vi "ReadPAQdata.vi"(4 "Tags":string[](array[string]), 6 "TableName":string, 8 "error in (no error)":errorcluster, 9 "Time-End":timestamp, 10 "Time-Start":timestamp, 11 "DBAL-BIN in":refnum<class "DBAL-BIN.lvclass">) -> (0 "error out":errorcluster, 2 "PAQ_section":T1, 3 "DBAL-BIN out":refnum<class "DBAL-BIN.lvclass">)   [LabVIEW 2020, in "Sgraph_lib_V1.lvlib" / "DBAL-BIN.lvclass"]
doc: "Andre Koelewijn, 8 May 2021,\n\nRead a PAQ TAGs from the BIN database for a defined time span.\nThe Layer input defines from which layer the data should be read.\nRev 1, 16 nov 2021, fixed gap when passing a day (midnight)"
uses:
  DBAL-BIN.lvclass
  controls/BIN/BINdata.ctl
  DBAL-BIN.lvclass/DBAL-BIN.ctl
  Gview/Gviewer.lvclass
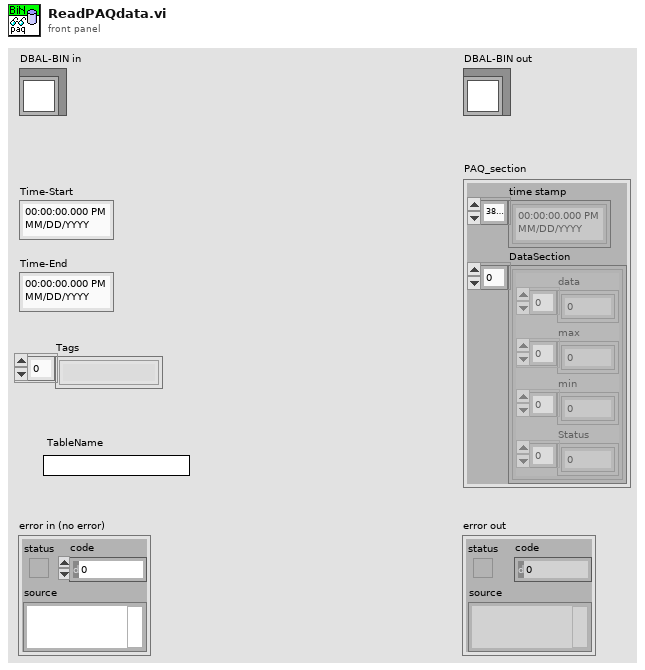
[diagram p1: front panel]
types:
  T1 = cluster{"time stamp":timestamp[], "DataSection":cluster{"data":dbl[], "max":dbl[], "min":dbl[], "Status":u32[]}[]}
  T2 = typedef "Sgraph_lib_V1.lvlib/DBAL-BIN.lvclass/BINdata.ctl" = cluster{"time":dbl[], "TagsData":cluster{"data":dbl[], "max":dbl[], "min":dbl[], "status":u32[]}[]}
  T3 = typedef "Sgraph_lib_V1.lvlib/DBAL-BIN.lvclass/BinFolderPace.ctl" = enum16{"PerDay", "PerWeek", "PerYear"}
  T4 = cluster{"Seq":i32, "Start":timestamp, "Stop":timestamp, "table":string}[]
  T5 = cluster{"data":dbl[], "max":dbl[], "min":dbl[], "status":u32[]}[]
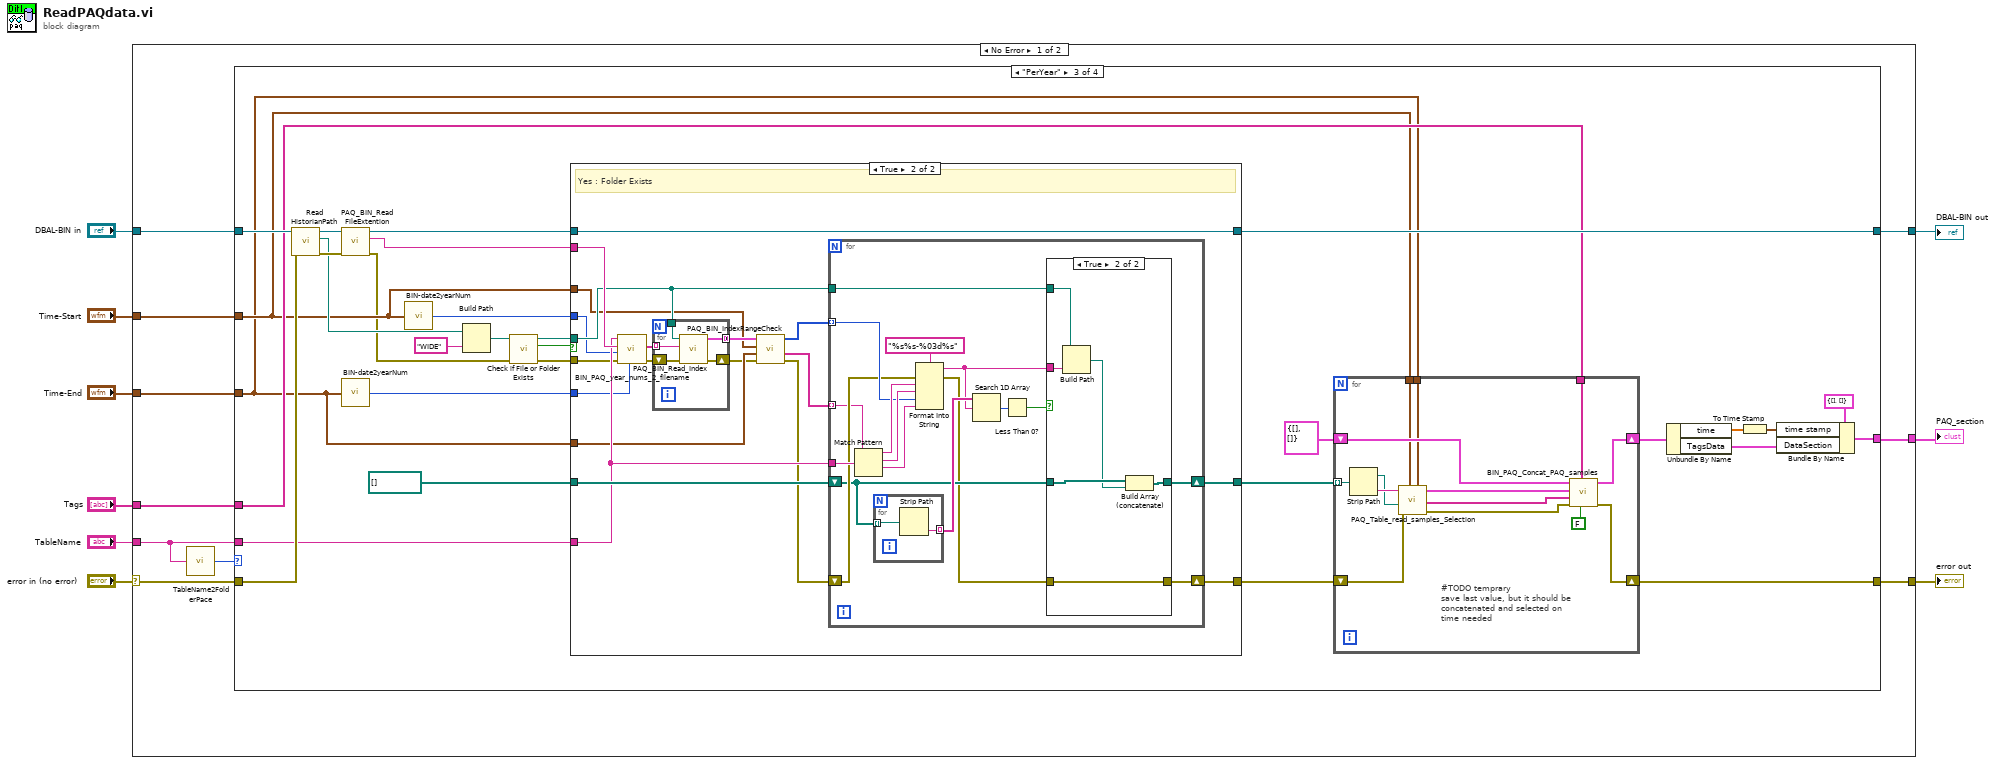
[diagram p0: block diagram]
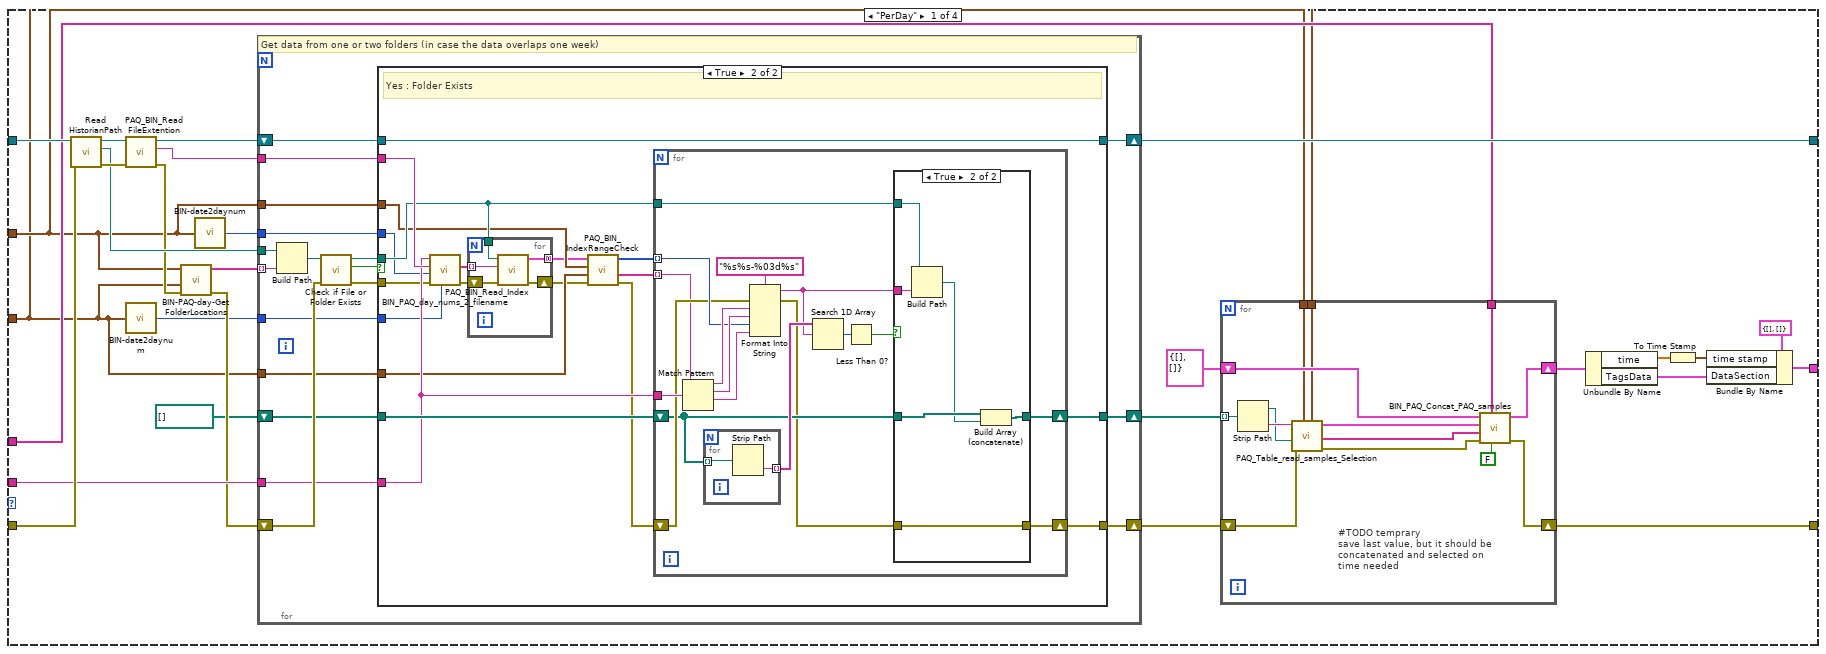
[diagram p2: hidden frame]
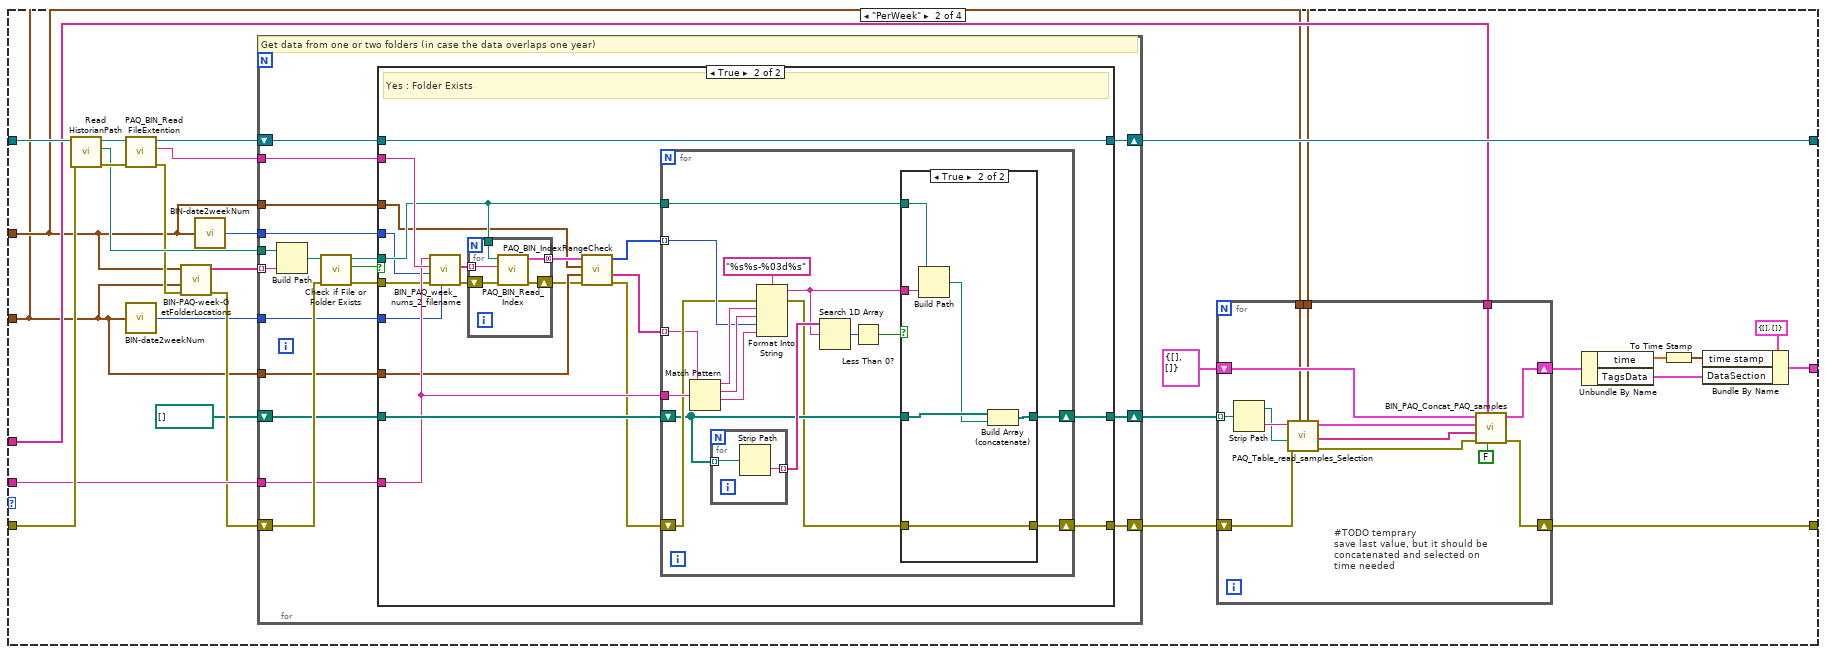
[diagram p5: hidden frame]
diagram:
  n1 = case shown="No Error" "error in (no error)" {
    selector: "error in (no error)" -> [w16 w350]
    tunnel: [w15 w350] -> w8
    tunnel: [w17 w349] -> w6
    tunnel: "DBAL-BIN in" -> [w18 w349]
    tunnel: "Time-Start" -> [w13 _]
    tunnel: "Time-End" -> [w12 _]
    tunnel: "Tags" -> [w11 _]
    tunnel: "TableName" -> [w14 _]
    tunnel: [w10 _] -> w1
    frame No Error {
      n2 = call "TableName2FolderPace.vi"("TableName"=w14) -> ("FolderPace"=w19:T3)  [unwired: 6 in]
      n3 = case shown="\"PerYear\"" w19 {
        tunnel: w18 -> [w47 w161 w278 w348]
        tunnel: [w42 w156 w273 w348] -> w17
        tunnel: w16 -> [w44 w158 w275 w347]
        tunnel: [w30 w144 w264 w347] -> w15
        tunnel: w14 -> [w41 w155 w272 _]
        tunnel: w13 -> [w21 w135 w255 _]
        tunnel: w12 -> [w20 w134 w254 _]
        tunnel: w11 -> [w22 w136 w256 _]
        tunnel: [w23 w137 w257 _] -> w10
        frame "PerDay" {
          n4 = call "Read HistorianPath.vi"("error in (no error)"=w44, "DBAL-BIN in"=w47) -> ("error out"=w45:errorcluster, "HistorianPath"=w39:path, "DBAL-BIN out"=w46:refnum<class "DBAL-BIN.lvclass">)  [unwired: 7 in]
          n5 = call "PAQ_BIN_Read FileExtention.vi"("error in (no error)"=w45, "DBAL-BIN in"=w46) -> ("error out"=w38:errorcluster, "FileExtention"=w40:string, "DBAL-BIN out"=w43:refnum<class "DBAL-BIN.lvclass">)  [unwired: 7 in]
          n6 = call "BIN-date2daynum.vi"("Time"=w20) -> ("DayNum"=w33:u64)  [unwired: 8 in]
          n7 = call "BIN-PAQ-day-GetFolderLocations.vi"("error in (no error)"=w38, "Time-End"=w20, "Time-Start"=w21) -> ("error out"=w36:errorcluster, "Folders"=w37:string[])  [unwired: 6 in, 1 out]
          n8 = call "BIN-date2daynum.vi"("Time"=w21) -> ("DayNum"=w32:u64)  [unwired: 8 in]
          n9 = for {
            shift-right: [w72] -> w31
            shift-left: w36 -> [w76]
            shift-right: [w73] -> w42
            shift-left: w43 -> [w74]
            tunnel: w37 -> [w78] mode=indexing
            tunnel: w41 -> [w66]
            tunnel: w39 -> [w79]
            tunnel: w40 -> [w71]
            shift-right: [w68] -> w34
            shift-left: path[] [] -> [w67]
            tunnel: w33 -> [w64]
            tunnel: w32 -> [w65]
            tunnel: w21 -> [w63]
            tunnel: w20 -> [w62]
            # "Get data from one or two folders (in case the data overlaps one week)"
            n10 = Build Path(base path=w79, name or relative path=w78) -> (appended path=w77:path)
            n11 = call <vilib>:"Check if File or Folder Exists.vi"("error in (no error)"=w76, "path"=w77) -> ("error out"=w69:errorcluster, "file or folder exists?"=w75:bool, "dup path"=w70:path)  [unwired: 7 in]
            n12 = case shown="True" w75 {
              tunnel: w74 -> [w82 w100]
              tunnel: [w82 w100] -> w73
              tunnel: [w81 w99] -> w72
              tunnel: w71 -> [_ w101]
              tunnel: w70 -> [_ w95]
              tunnel: w69 -> [w81 w93]
              tunnel: [w80 w97] -> w68
              tunnel: w67 -> [w80 w98]
              tunnel: w66 -> [_ w96]
              tunnel: w65 -> [_ w92]
              tunnel: w64 -> [_ w91]
              tunnel: w63 -> [_ w89]
              tunnel: w62 -> [_ w88]
              frame False {
                # "No: Folder not found"
              }
              frame True {
                # "Yes : Folder Exists"
                n13 = call "BIN_PAQ_day_nums_2_filename.vi"("num Stop"=w91, "error in"=w93, "num Start"=w92, "ext"=w101, "TableName"=w96) -> ("error out"=w94:errorcluster, "FileNames"=w90:string[])  [unwired: 5 in]
                n14 = for {
                  tunnel: [w106] -> w87 mode=concatenating
                  tunnel: w95 -> [w104]
                  shift-right: [w105] -> w84
                  shift-left: w94 -> [w103]
                  tunnel: w90 -> [w102] mode=indexing
                  n15 = call "PAQ_BIN_Read_Index.vi"("error in (no error)"=w103, "TableName"=w102, "Path"=w104) -> ("error out"=w105:errorcluster, "TimeStamps"=w106:T4)  [unwired: 7 in]
                }
                n16 = call "PAQ_BIN_IndexRangeCheck.vi"("error in (no error)"=w84, "Stop"=w88, "Start"=w89, "TimeStamps"=w87) -> ("error out"=w83:errorcluster, "Tables"=w85:string[], "Sequences"=w86:i32[])  [unwired: 5 in]
                n17 = for {
                  shift-right: [w108] -> w99
                  shift-left: w83 -> [w116]
                  tunnel: w86 -> [w119] mode=indexing
                  shift-right: [w110] -> w97
                  shift-left: w98 -> [w111]
                  tunnel: w96 -> [w123]
                  tunnel: w95 -> [w112]
                  tunnel: w85 -> [w107] mode=indexing
                  n18 = Match Pattern(string=w107, regular expression=w123) -> (before substring=w121:string, match substring=w120:string, after substring=w118:string)  [unwired: 1 in, 1 out]
                  n19 = for {
                    tunnel: w111 -> [w133] mode=indexing
                    tunnel: [w132] -> w117 mode=indexing
                    n20 = Strip Path(path=w133) -> (name=w132:string)  [unwired: 1 out]
                  }
                  n21 = Format Into String(format string="%s%s-%03d%s", error in=w116, w121, w120, w119, w118) -> (resulting string=w113:string, error out=w109:errorcluster)  [unwired: 1 in]
                  n22 = Search 1D Array(1D array=w117, element=w113) -> (index of element=w115:i32)  [unwired: 1 in]
                  n23 = Less Than 0?(x=w115) -> (x < 0?=w114:bool)
                  n24 = case shown="True" w114 {
                    tunnel: w113 -> [_ w130]
                    tunnel: w112 -> [_ w131]
                    tunnel: w111 -> [w125 w127]
                    tunnel: [w125 w128] -> w110
                    tunnel: w109 -> [w124 w129]
                    tunnel: [w124 w129] -> w108
                    frame False {
                    }
                    frame True {
                      n25 = Build Path(base path=w131, name or relative path=w130) -> (appended path=w126:path)
                      n26 = Build Array (concatenate)(w127, w126) -> (w128:path[])
                    }
                  }
                }
              }
            }
          }
          n27 = for {
            tunnel: w34 -> [w60] mode=indexing
            shift-right: [w51] -> w30
            shift-left: w31 -> [w61]
            shift-right: [w56] -> w24
            shift-left: T2 {"time"=[], "TagsData"=[]} ("BinHistData") -> [w57]
            tunnel: w22 -> [w54]
            tunnel: w21 -> [w50]
            tunnel: w20 -> [w49]
            # "#TODO temprary\nsave last value, but it should be\nconcatenated and selected on \ntime needed"
            n28 = Strip Path(path=w60) -> (stripped path=w58:path, name=w59:string)
            n29 = call "PAQ_Table_read_samples_Selection.vi"("Time-End"=w49, "Time-Start"=w50, "error in (no error)"=w61, "Sub Path"=w58, "Table Filename"=w59) -> ("error out"=w52:errorcluster, "TAGs"=w53:string[], "Fetched PAQ-samples"=w55:T2)  [unwired: 3 in, 1 out]
            n30 = call "BIN_PAQ_Concat_PAQ_samples.vi"("Reversed"=FALSE, "Memory TAGs"=w54, "error in (no error)"=w52, "Added samples TAGs"=w53, "PAQ Samples to ADD"=w55, "PAQ Samples IN"=w57) -> ("error out"=w51:errorcluster, "PAQ Samples OUT"=w56:T2)  [unwired: 4 in]
          }
          n31 = Unbundle By Name(w24) -> ("time"=w27:dbl[], "TagsData"=w28:T5)
          n32 = To Time Stamp(1:w27) -> (0:w26:timestamp[])
          n33 = Bundle By Name(cluster=T1 {"time stamp"=[], "DataSection"=[]} ("PAQ_section"), "time stamp"=w26, "DataSection"=w28) -> (w23:T1)
        }
        frame "PerWeek" {
          n34 = call "Read HistorianPath.vi"("error in (no error)"=w158, "DBAL-BIN in"=w161) -> ("error out"=w159:errorcluster, "HistorianPath"=w153:path, "DBAL-BIN out"=w160:refnum<class "DBAL-BIN.lvclass">)  [unwired: 7 in]
          n35 = call "PAQ_BIN_Read FileExtention.vi"("error in (no error)"=w159, "DBAL-BIN in"=w160) -> ("error out"=w152:errorcluster, "FileExtention"=w154:string, "DBAL-BIN out"=w157:refnum<class "DBAL-BIN.lvclass">)  [unwired: 7 in]
          n36 = call "BIN-date2weekNum.vi"("Time"=w134) -> ("WeekNum"=w147:u64)  [unwired: 8 in]
          n37 = call "BIN-PAQ-week-GetFolderLocations.vi"("error in (no error)"=w152, "Time-End"=w134, "Time-Start"=w135) -> ("error out"=w150:errorcluster, "Folders"=w151:string[])  [unwired: 6 in, 1 out]
          n38 = call "BIN-date2weekNum.vi"("Time"=w135) -> ("WeekNum"=w146:u64)  [unwired: 8 in]
          n39 = for {
            shift-right: [w186] -> w145
            shift-left: w150 -> [w190]
            shift-right: [w187] -> w156
            shift-left: w157 -> [w188]
            tunnel: w151 -> [w192] mode=indexing
            tunnel: w155 -> [w180]
            tunnel: w153 -> [w193]
            tunnel: w154 -> [w185]
            shift-right: [w182] -> w148
            shift-left: path[] [] -> [w181]
            tunnel: w147 -> [w178]
            tunnel: w146 -> [w179]
            tunnel: w135 -> [w177]
            tunnel: w134 -> [w176]
            # "Get data from one or two folders (in case the data overlaps one year)"
            n40 = Build Path(base path=w193, name or relative path=w192) -> (appended path=w191:path)
            n41 = call <vilib>:"Check if File or Folder Exists.vi"("error in (no error)"=w190, "path"=w191) -> ("error out"=w183:errorcluster, "file or folder exists?"=w189:bool, "dup path"=w184:path)  [unwired: 7 in]
            n42 = case shown="True" w189 {
              tunnel: w188 -> [w196 w214]
              tunnel: [w196 w214] -> w187
              tunnel: [w195 w213] -> w186
              tunnel: w185 -> [_ w215]
              tunnel: w184 -> [_ w209]
              tunnel: w183 -> [w195 w207]
              tunnel: [w194 w211] -> w182
              tunnel: w181 -> [w194 w212]
              tunnel: w180 -> [_ w210]
              tunnel: w179 -> [_ w206]
              tunnel: w178 -> [_ w205]
              tunnel: w177 -> [_ w202]
              tunnel: w176 -> [_ w201]
              frame False {
                # "No: Folder not found"
              }
              frame True {
                # "Yes : Folder Exists"
                n43 = call "BIN_PAQ_week_nums_2_filename.vi"("num Stop"=w205, "error in"=w207, "num Start"=w206, "ext"=w215, "TableName"=w210) -> ("error out"=w208:errorcluster, "FileNames"=w204:string[])  [unwired: 5 in]
                n44 = for {
                  tunnel: [w220] -> w203 mode=concatenating
                  tunnel: w209 -> [w218]
                  shift-right: [w219] -> w200
                  shift-left: w208 -> [w217]
                  tunnel: w204 -> [w216] mode=indexing
                  n45 = call "PAQ_BIN_Read_Index.vi"("error in (no error)"=w217, "TableName"=w216, "Path"=w218) -> ("error out"=w219:errorcluster, "TimeStamps"=w220:T4)  [unwired: 7 in]
                }
                n46 = call "PAQ_BIN_IndexRangeCheck.vi"("error in (no error)"=w200, "Stop"=w201, "Start"=w202, "TimeStamps"=w203) -> ("error out"=w199:errorcluster, "Tables"=w197:string[], "Sequences"=w198:i32[])  [unwired: 5 in]
                n47 = for {
                  shift-right: [w222] -> w213
                  shift-left: w199 -> [w230]
                  tunnel: w198 -> [w233] mode=indexing
                  shift-right: [w224] -> w211
                  shift-left: w212 -> [w225]
                  tunnel: w210 -> [w237]
                  tunnel: w209 -> [w226]
                  tunnel: w197 -> [w221] mode=indexing
                  n48 = Match Pattern(string=w221, regular expression=w237) -> (before substring=w235:string, match substring=w234:string, after substring=w232:string)  [unwired: 1 in, 1 out]
                  n49 = for {
                    tunnel: w225 -> [w247] mode=indexing
                    tunnel: [w246] -> w231 mode=indexing
                    n50 = Strip Path(path=w247) -> (name=w246:string)  [unwired: 1 out]
                  }
                  n51 = Format Into String(format string="%s%s-%03d%s", error in=w230, w235, w234, w233, w232) -> (resulting string=w227:string, error out=w223:errorcluster)  [unwired: 1 in]
                  n52 = Search 1D Array(1D array=w231, element=w227) -> (index of element=w229:i32)  [unwired: 1 in]
                  n53 = Less Than 0?(x=w229) -> (x < 0?=w228:bool)
                  n54 = case shown="True" w228 {
                    tunnel: w227 -> [_ w244]
                    tunnel: w226 -> [_ w245]
                    tunnel: w225 -> [w239 w242]
                    tunnel: [w239 w240] -> w224
                    tunnel: w223 -> [w238 w243]
                    tunnel: [w238 w243] -> w222
                    frame False {
                    }
                    frame True {
                      n55 = Build Path(base path=w245, name or relative path=w244) -> (appended path=w241:path)
                      n56 = Build Array (concatenate)(w242, w241) -> (w240:path[])
                    }
                  }
                }
              }
            }
          }
          n57 = for {
            tunnel: w148 -> [w174] mode=indexing
            shift-right: [w165] -> w144
            shift-left: w145 -> [w175]
            shift-right: [w170] -> w138
            shift-left: T2 {"time"=[], "TagsData"=[]} ("BinHistData") -> [w171]
            tunnel: w136 -> [w168]
            tunnel: w135 -> [w164]
            tunnel: w134 -> [w163]
            # "#TODO temprary\nsave last value, but it should be\nconcatenated and selected on \ntime needed"
            n58 = Strip Path(path=w174) -> (stripped path=w172:path, name=w173:string)
            n59 = call "PAQ_Table_read_samples_Selection.vi"("Time-End"=w163, "Time-Start"=w164, "error in (no error)"=w175, "Sub Path"=w172, "Table Filename"=w173) -> ("error out"=w166:errorcluster, "TAGs"=w167:string[], "Fetched PAQ-samples"=w169:T2)  [unwired: 3 in, 1 out]
            n60 = call "BIN_PAQ_Concat_PAQ_samples.vi"("Reversed"=FALSE, "Memory TAGs"=w168, "error in (no error)"=w166, "Added samples TAGs"=w167, "PAQ Samples to ADD"=w169, "PAQ Samples IN"=w171) -> ("error out"=w165:errorcluster, "PAQ Samples OUT"=w170:T2)  [unwired: 4 in]
          }
          n61 = Unbundle By Name(w138) -> ("time"=w141:dbl[], "TagsData"=w142:T5)
          n62 = To Time Stamp(1:w141) -> (0:w140:timestamp[])
          n63 = Bundle By Name(cluster=T1 {"time stamp"=[], "DataSection"=[]} ("PAQ_section"), "time stamp"=w140, "DataSection"=w142) -> (w137:T1)
        }
        frame "PerYear" {
          n64 = call "Read HistorianPath.vi"("error in (no error)"=w275, "DBAL-BIN in"=w278) -> ("error out"=w276:errorcluster, "HistorianPath"=w270:path, "DBAL-BIN out"=w277:refnum<class "DBAL-BIN.lvclass">)  [unwired: 7 in]
          n65 = call "PAQ_BIN_Read FileExtention.vi"("error in (no error)"=w276, "DBAL-BIN in"=w277) -> ("error out"=w253:errorcluster, "FileExtention"=w271:string, "DBAL-BIN out"=w274:refnum<class "DBAL-BIN.lvclass">)  [unwired: 7 in]
          n66 = call "BIN-date2yearNum.vi"("Time"=w254) -> ("YearNum"=w267:u64)  [unwired: 8 in]
          n67 = call "BIN-date2yearNum.vi"("Time"=w255) -> ("YearNum"=w266:u64)  [unwired: 8 in]
          n68 = Build Path(base path=w270, name or relative path="WIDE") -> (appended path=w252:path)
          n69 = call <vilib>:"Check if File or Folder Exists.vi"("error in (no error)"=w253, "path"=w252) -> ("error out"=w249:errorcluster, "file or folder exists?"=w251:bool, "dup path"=w250:path)  [unwired: 7 in]
          n70 = case shown="True" w251 {
            tunnel: w274 -> [w281 w299]
            tunnel: [w281 w299] -> w273
            tunnel: [w280 w298] -> w265
            tunnel: w271 -> [_ w300]
            tunnel: w250 -> [_ w294]
            tunnel: w249 -> [w280 w292]
            tunnel: [w279 w296] -> w268
            tunnel: path[] [] -> [w279 w297]
            tunnel: w272 -> [_ w295]
            tunnel: w266 -> [_ w291]
            tunnel: w267 -> [_ w290]
            tunnel: w255 -> [_ w287]
            tunnel: w254 -> [_ w286]
            frame False {
              # "No: Folder not found"
            }
            frame True {
              # "Yes : Folder Exists"
              n71 = call "BIN_PAQ_year_nums_2_filename.vi"("num Stop"=w290, "error in"=w292, "num Start"=w291, "ext"=w300, "TableName"=w295) -> ("error out"=w293:errorcluster, "FileNames"=w289:string[])  [unwired: 5 in]
              n72 = for {
                tunnel: [w305] -> w288 mode=concatenating
                tunnel: w294 -> [w303]
                shift-right: [w304] -> w285
                shift-left: w293 -> [w302]
                tunnel: w289 -> [w301] mode=indexing
                n73 = call "PAQ_BIN_Read_Index.vi"("error in (no error)"=w302, "TableName"=w301, "Path"=w303) -> ("error out"=w304:errorcluster, "TimeStamps"=w305:T4)  [unwired: 7 in]
              }
              n74 = call "PAQ_BIN_IndexRangeCheck.vi"("error in (no error)"=w285, "Stop"=w286, "Start"=w287, "TimeStamps"=w288) -> ("error out"=w284:errorcluster, "Tables"=w282:string[], "Sequences"=w283:i32[])  [unwired: 5 in]
              n75 = for {
                shift-right: [w307] -> w298
                shift-left: w284 -> [w315]
                tunnel: w283 -> [w318] mode=indexing
                shift-right: [w309] -> w296
                shift-left: w297 -> [w310]
                tunnel: w295 -> [w322]
                tunnel: w294 -> [w311]
                tunnel: w282 -> [w306] mode=indexing
                n76 = Match Pattern(string=w306, regular expression=w322) -> (before substring=w320:string, match substring=w319:string, after substring=w317:string)  [unwired: 1 in, 1 out]
                n77 = for {
                  tunnel: w310 -> [w332] mode=indexing
                  tunnel: [w331] -> w316 mode=indexing
                  n78 = Strip Path(path=w332) -> (name=w331:string)  [unwired: 1 out]
                }
                n79 = Format Into String(format string="%s%s-%03d%s", error in=w315, w320, w319, w318, w317) -> (resulting string=w312:string, error out=w308:errorcluster)  [unwired: 1 in]
                n80 = Search 1D Array(1D array=w316, element=w312) -> (index of element=w314:i32)  [unwired: 1 in]
                n81 = Less Than 0?(x=w314) -> (x < 0?=w313:bool)
                n82 = case shown="True" w313 {
                  tunnel: w312 -> [_ w329]
                  tunnel: w311 -> [_ w330]
                  tunnel: w310 -> [w324 w327]
                  tunnel: [w324 w325] -> w309
                  tunnel: w308 -> [w323 w328]
                  tunnel: [w323 w328] -> w307
                  frame False {
                  }
                  frame True {
                    n83 = Build Path(base path=w330, name or relative path=w329) -> (appended path=w326:path)
                    n84 = Build Array (concatenate)(w327, w326) -> (w325:path[])
                  }
                }
              }
            }
          }
          n85 = for {
            tunnel: w268 -> [w345] mode=indexing
            shift-right: [w336] -> w264
            shift-left: w265 -> [w346]
            shift-right: [w341] -> w258
            shift-left: T2 {"time"=[], "TagsData"=[]} ("BinHistData") -> [w342]
            tunnel: w256 -> [w339]
            tunnel: w255 -> [w335]
            tunnel: w254 -> [w334]
            # "#TODO temprary\nsave last value, but it should be\nconcatenated and selected on \ntime needed"
            n86 = Strip Path(path=w345) -> (stripped path=w343:path, name=w344:string)
            n87 = call "PAQ_Table_read_samples_Selection.vi"("Time-End"=w334, "Time-Start"=w335, "error in (no error)"=w346, "Sub Path"=w343, "Table Filename"=w344) -> ("error out"=w337:errorcluster, "TAGs"=w338:string[], "Fetched PAQ-samples"=w340:T2)  [unwired: 3 in, 1 out]
            n88 = call "BIN_PAQ_Concat_PAQ_samples.vi"("Reversed"=FALSE, "Memory TAGs"=w339, "error in (no error)"=w337, "Added samples TAGs"=w338, "PAQ Samples to ADD"=w340, "PAQ Samples IN"=w342) -> ("error out"=w336:errorcluster, "PAQ Samples OUT"=w341:T2)  [unwired: 4 in]
          }
          n89 = Unbundle By Name(w258) -> ("time"=w261:dbl[], "TagsData"=w262:T5)
          n90 = To Time Stamp(1:w261) -> (0:w260:timestamp[])
          n91 = Bundle By Name(cluster=T1 {"time stamp"=[], "DataSection"=[]} ("PAQ_section"), "time stamp"=w260, "DataSection"=w262) -> (w257:T1)
        }
        frame Default {
        }
      }
    }
    frame Error {
    }
  }
  "error out" <- w8
  "DBAL-BIN out" <- w6
  "PAQ_section" <- w1
